vi "get full seq channel list.vi"(11 "engine configuration in":refnum<class "base TBM sequencer configuration.lvclass">) -> (2 "seq channel list":refnum<class "TBM channel.lvclass">[](array[class]), 3 "engine configuration out":refnum<class "base TBM sequencer configuration.lvclass">)   [LabVIEW 2014, in "base TBM sequencer configuration.lvclass"]
uses:
  base TBM sequencer configuration.lvclass
  <vilib>/NI/Tag Bus Module Framework/channel/TBM channel.lvclass
  base TBM sequencer configuration.lvclass/base TBM sequencer configuration.ctl
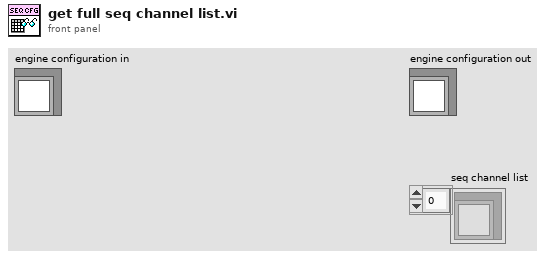
[diagram p1: front panel]
types:
  T1 = typedef "base TBM sequencer configuration.lvclass/Tag Info.ctl" = cluster{"Channel":refnum<class "TBM channel.lvclass">, "Writers":string[], "Readers":string[], "Owning ID":string}
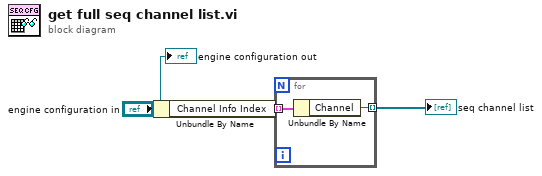
[diagram p0: block diagram]
diagram:
  n1 = Unbundle By Name("engine configuration in") -> ("Channel Info Index"=w3:T1[])
  n2 = for {
    tunnel: w3 -> [w5] mode=indexing
    tunnel: [w4] -> w2 mode=indexing
    n3 = Unbundle By Name(w5) -> ("Channel"=w4:refnum<class "TBM channel.lvclass">)
  }
  "seq channel list" <- w2
  "engine configuration out" <- "engine configuration in"
